vi "TSM Digital Initialize Sessions.vi"(0 "TSM context":T1) -> (15 "error out":errorcluster)   [LabVIEW 2020]
doc: "Use this VI to initialize sessions for all NI-Digital Pattern instruments in the pin map associated with the test program and apply an initial level and timing sheet to these instruments."
uses:
  <vilib>/NI_TestStand_SemiconductorModule/NI_TestStand_Semiconductor_Module.lvlibp/PinMap/General/SemiconductorModuleContext.ctl
  <instrlib>/niDigital/niDigital.llb/niDigital Load Specifications Levels and Timing (Multiple).vi
  <instrlib>/niDigital/niDigital.llb/niDigital Create Capture Waveform From File (Digicapture).vi
  <instrlib>/niDigital/niDigital.llb/niDigital Create Source Waveform From File (TDMS).vi
  <vilib>/NI_TestStand_SemiconductorModule/NI_TestStand_Semiconductor_Module.lvlibp
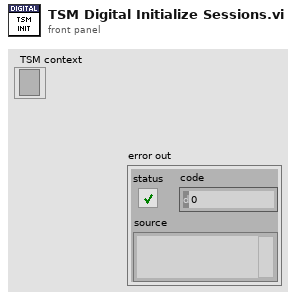
[diagram p1: front panel]
types:
  T1 = typedef "NI_TestStand_Semiconductor_Module.lvlibp/SemiconductorModuleContext.ctl" = refnum<k7>
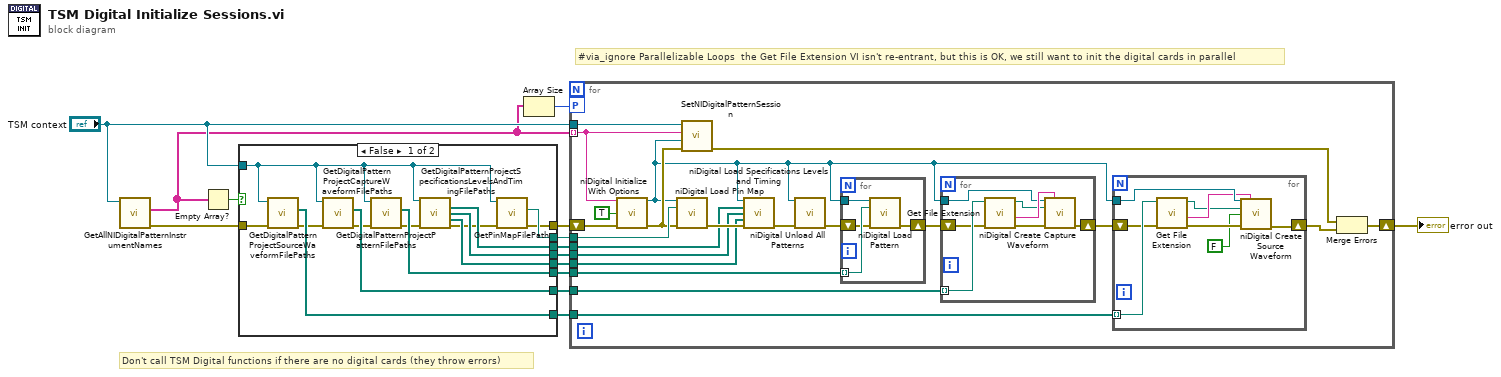
[diagram p0: block diagram]
diagram:
  # "Don't call TSM Digital functions if there are no digital cards (they throw errors)"
  # "#via_ignore Parallelizable Loops  the Get File Extension VI isn't re-entrant, but this is OK, we still want to init the digital cards in parallel"
  n1 = call <vilib>:"GetAllNIDigitalPatternInstrumentNames.vi"("Semiconductor Module Context"="TSM context") -> ("error out"=w6:errorcluster, "Instrument Names"=w2:string[])  [unwired: 8 in, 1 out]
  n2 = Empty Array?(array=w2) -> (empty?=w1:bool)
  n3 = case shown="False" w1 {
    tunnel: [w28 _] -> w14
    tunnel: [w27 _] -> w13
    tunnel: [w26 _] -> w12
    tunnel: [w25 _] -> w11
    tunnel: [w24 _] -> w10
    tunnel: [w22 w29] -> w9
    tunnel: [w20 _] -> w8
    tunnel: [w19 _] -> w7
    tunnel: w6 -> [w18 w29]
    tunnel: "TSM context" -> [w15 _]
    frame False {
      n4 = call <vilib>:"GetDigitalPatternProjectSourceWaveformFilePaths.vi"("error in (no error)"=w18, "Semiconductor Module Context"=w15) -> ("error out"=w17:errorcluster, "Source Waveform File Paths"=w19:path[])  [unwired: 7 in, 1 out]
      n5 = call <vilib>:"GetDigitalPatternProjectCaptureWaveformFilePaths.vi"("error in (no error)"=w17, "Semiconductor Module Context"=w15) -> ("error out"=w16:errorcluster, "Capture Waveform File Paths"=w20:path[])  [unwired: 7 in, 1 out]
      n6 = call <vilib>:"GetDigitalPatternProjectPatternFilePaths.vi"("error in (no error)"=w16, "Semiconductor Module Context"=w15) -> ("error out"=w21:errorcluster, "Pattern File Paths"=w24:path[])  [unwired: 7 in, 1 out]
      n7 = call <vilib>:"GetDigitalPatternProjectSpecificationsLevelsAndTimingFilePaths.vi"("Semiconductor Module Context"=w15, "error in (no error)"=w21) -> ("Specifications File Paths"=w27:path[], "Levels File Paths"=w26:path[], "Timing File Paths"=w25:path[], "error out"=w23:errorcluster)  [unwired: 9 in, 1 out]
      n8 = call <vilib>:"GetPinMapFilePath.vi"("error in (no error)"=w23, "Semiconductor Module Context"=w15) -> ("error out"=w22:errorcluster, "Pin Map File Path"=w28:path)  [unwired: 7 in, 1 out]
    }
    frame True {
    }
  }
  n9 = Array Size(array=w2) -> (size(s)=w4:i32)
  n10 = for {
    tunnel: w2 -> [w48] mode=indexing
    tunnel: "TSM context" -> [w42]
    tunnel: w14 -> [w46]
    tunnel: w13 -> [w45]
    tunnel: w12 -> [w44]
    tunnel: w11 -> [w43]
    tunnel: w8 -> [w40]
    tunnel: w10 -> [w41]
    tunnel: w7 -> [w39]
    shift-right: [w33] -> w5
    shift-left: w9 -> [w50]
    workers-P: w4 -> [_]
    n11 = call <instrlib>:"niDigital Initialize With Options.vi"("resource name"=w48, "reset (T)"=TRUE, "error in"=w50) -> ("instrument handle"=w30:refnum<k15>, "error out"=w34:errorcluster)  [unwired: 11 in]
    n12 = call <instrlib>:"niDigital Load Pin Map.vi"("instrument handle"=w30, "pin map file"=w46, "error in"=w34) -> ("error out"=w49:errorcluster)  [unwired: 11 in, 1 out]
    n13 = call <vilib>:"SetNIDigitalPatternSession.vi"("error in (no error)"=w34, "Instrument Session"=w30, "Instrument Name"=w48, "Semiconductor Module Context"=w42) -> ("error out"=w31:errorcluster)  [unwired: 6 in, 1 out]
    n14 = call-poly <instrlib>:"niDigital Load Specifications Levels and Timing.vi"("instrument handle"=w30, "specifications file paths"=w45, "levels file paths"=w44, "timing file paths"=w43, "error in"=w49) -> ("error out"=w35:errorcluster)  [unwired: 9 in, 1 out]
    n15 = call <instrlib>:"niDigital Unload All Patterns.vi"("instrument handle"=w30, "error in"=w35) -> ("error out"=w37:errorcluster)  [unwired: 12 in, 1 out]
    n16 = for {
      tunnel: w41 -> [w67] mode=indexing
      shift-right: [w69] -> w36
      shift-left: w37 -> [w66]
      tunnel: w30 -> [w68]
      n17 = call <instrlib>:"niDigital Load Pattern.vi"("instrument handle"=w68, "pattern file"=w67, "error in"=w66) -> ("error out"=w69:errorcluster)  [unwired: 11 in, 1 out]
    }
    n18 = for {
      tunnel: w40 -> [w62] mode=indexing
      shift-right: [w61] -> w38
      shift-left: w36 -> [w59]
      tunnel: w30 -> [w60]
      n19 = call <vilib>:"Get File Extension.vi"("error in (no error)"=w59, "file"=w62) -> ("error out"=w65:errorcluster, "filename without extension"=w64:string, "dup file"=w63:path)  [unwired: 5 in, 2 out]
      n20 = call-poly <instrlib>:"niDigital Create Capture Waveform.vi"("instrument handle"=w60, "waveform name"=w64, "waveform file"=w63, "error in"=w65) -> ("error out"=w61:errorcluster)  [unwired: 10 in, 1 out]
    }
    n21 = for {
      tunnel: w39 -> [w53] mode=indexing
      shift-right: [w51] -> w32
      shift-left: w38 -> [w52]
      tunnel: w30 -> [w57]
      n22 = call <vilib>:"Get File Extension.vi"("error in (no error)"=w52, "file"=w53) -> ("error out"=w58:errorcluster, "filename without extension"=w56:string, "dup file"=w55:path)  [unwired: 5 in, 2 out]
      n23 = call-poly <instrlib>:"niDigital Create Source Waveform.vi"("instrument handle"=w57, "waveform name"=w56, "waveform file"=w55, "write waveform data (T)"=FALSE, "error in"=w58) -> ("error out"=w51:errorcluster)  [unwired: 9 in, 1 out]
    }
    n24 = Merge Errors(w31, w32) -> (w33:errorcluster)
  }
  "error out" <- w5
